vi "PV Temperature info.vi"(0 "VISA session":refnum<visa-resource-name>, 5 "Adress of unit":u16=1 min=1 max=999 step=1, 7 "Parameter":T1(ring), 11 "error in (no error)":errorcluster) -> (4 "dup VISA session":refnum<visa-resource-name>, 6 "response (data)":string, 15 "error out":errorcluster)   [LabVIEW 2024, in "Pfeiffer Vacuum.lvlib"]
doc: "There are 6 parameters available, only one of which can be enabled at a time. \n\ntemperature inverter [°C] (default) (324)\ntemperature electronic [°C] (326)\ntemperature pump bottom [°C] (330)\ntemperature bearing [°C] (342)\ntemperature motor [°C] (346)\ntemperature rotor [°C] (384)\n\nNote: Any settings for an parameter that is not selected will be ignored. If a value is out of range, it will be changed to either the upper or the lower limit of the range."
uses:
  <instrlib>/Pfeiffer Vacuum/Pfeiffer Vacuum.lvlib
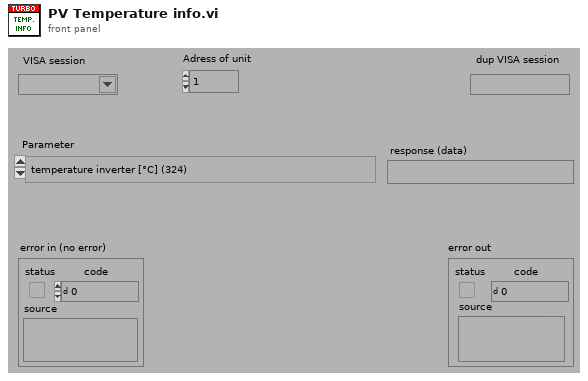
[diagram p1: front panel]
types:
  T1 = enum16{"temperature inverter [°C] (324)", "temperature electronic [°C] (326)", "temperature pump bottom [°C] (330)", "temperature bearing [°C] (342)", "temperature motor [°C] (346)", "temperature rotor [°C] (384)"}
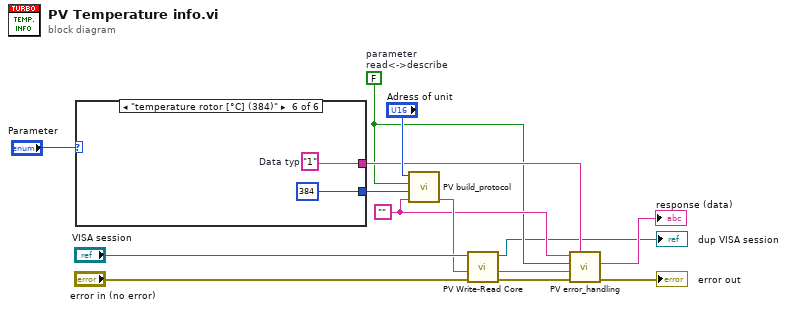
[diagram p0: block diagram]
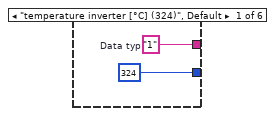
[diagram p2: hidden frame]
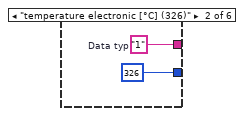
[diagram p3: hidden frame]
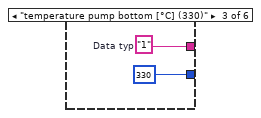
[diagram p4: hidden frame]
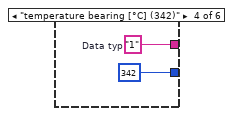
[diagram p5: hidden frame]
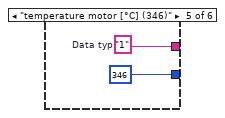
[diagram p6: hidden frame]
diagram:
  w7 = ""
  w6 = FALSE  # parameter read<->describe
  n1 = case shown="\"temperature rotor [°C] (384)\"" "Parameter" {
    tunnel: [u16 324 ("Parameter-number") u16 326 ("Parameter-number") u16 330 ("Parameter-number") u16 342 ("Parameter-number") u16 346 ("Parameter-number") u16 384 ("Parameter-number")] -> w12
    tunnel: [w15 w17 w19 w21 w24 w26] -> w8
    frame "temperature inverter [°C] (324)", Default {
      w15 = "1"  # Data typ
    }
    frame "temperature electronic [°C] (326)" {
      w17 = "1"  # Data typ
    }
    frame "temperature pump bottom [°C] (330)" {
      w19 = "1"  # Data typ
    }
    frame "temperature bearing [°C] (342)" {
      w21 = "1"  # Data typ
    }
    frame "temperature motor [°C] (346)" {
      w24 = "1"  # Data typ
    }
    frame "temperature rotor [°C] (384)" {
      w26 = "1"  # Data typ
    }
  }
  n2 = call <instrlib>:"PV build_protocol.vi"("Data"=w7, "Parameter-number"=w12, "parameter\nread<->describe"=w6, "Adress"="Adress of unit") -> ("output"=w9:string)  [unwired: 3 in]
  n3 = call <instrlib>:"PV Write-Read Core.vi"("error in"="error in (no error)", "Write data in"=w9, "VISA session"="VISA session") -> ("error out"=w4:errorcluster, "response (data) out"=w5:string, "dup VISA session"=→"dup VISA session":refnum<visa-resource-name>)  [unwired: 2 in]
  n4 = call <instrlib>:"PV error_handling.vi"("Data Typ in"=w8, "error in"=w4, "response (data) in"=w5, "Parameter\nread only<->describe"=w6, "data in"=w7) -> ("error out"=→"error out":errorcluster, "Data out"=→"response (data)":string)  [unwired: 4 in, 1 out]
